vi "H5Fget_name.vi"(6 "error in (no error)":errorcluster, 9 "HDF5 Attr Ref":T1) -> (0 "error out":errorcluster, 2 "Name":string, 3 "HDF5 Attr Ref out":T1)   [LabVIEW 2017]
doc: "Retrieves name of file to which object belongs."
uses:
  <vilib>/UPVI/lvhdf5/library.llb/HDF5 Ref.ctl
  <vilib>/UPVI/lvhdf5/hdf5.dll
panel:
  # "LVHDF5 Toolkit\nCopyright (c) 2005-2013 by Jason D. Sommerville\nCopyright (c) 2014 by UPVI, LLC.\n\nThis use and distribution of this file is governed by the terms found in \nLICENSE.txt distributed with this toolkit and installed at\n <user.lib>\\_lvhdf5\\LICENSE.txt"
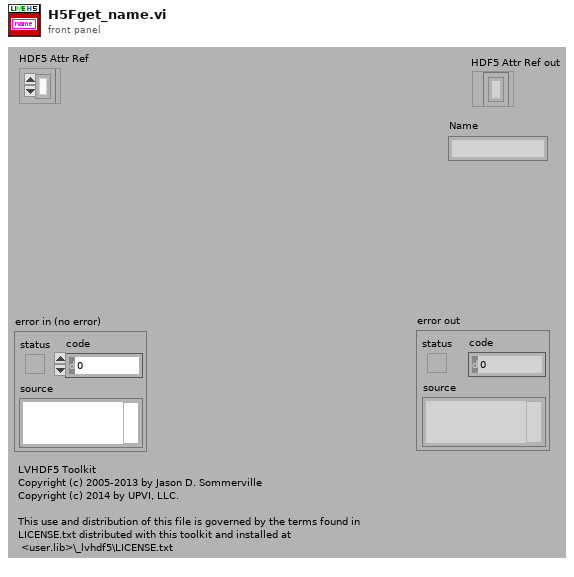
[diagram p1: front panel]
types:
  T1 = typedef "HDF5 Ref.ctl" = refnum<k1>
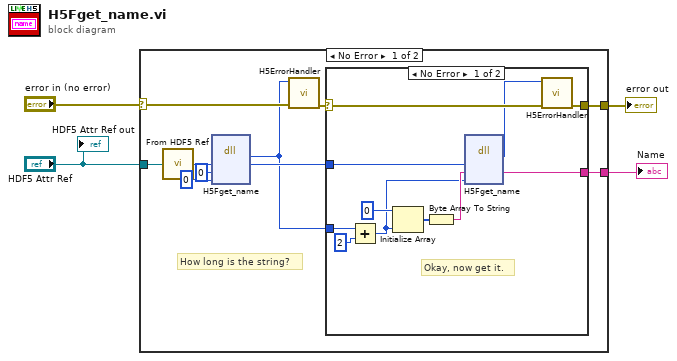
[diagram p0: block diagram]
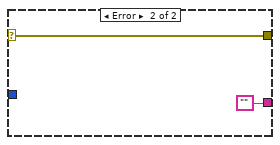
[diagram p2: hidden frame]
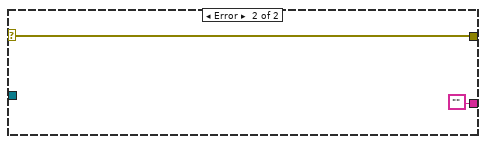
[diagram p3: hidden frame]
diagram:
  n1 = case shown="No Error" "error in (no error)" {
    selector: "error in (no error)" -> [w12 w29]
    tunnel: [w8 w29] -> w2
    tunnel: "HDF5 Attr Ref" -> [w14 _]
    tunnel: [w9 ""] -> w1
    frame No Error {
      # "How long is the string?"
      n2 = call <vilib>:"From HDF5 Ref.vi"("HDF5 Ref"=w14) -> ("I32"=w13:i32)
      n3 = dll-call lib="C:/Program Files/National Instruments/LabVIEW 2017/vi.lib/UPVI/lvhdf5/hdf5.dll" fn="H5Fget_name"("obj_id"=w13, "name"=0, "size"=u32 0) -> ("return type"=w7:u64, "obj_id"=w10:i32)  [unwired: 5 in, 2 out]
      n4 = call <vilib>:"H5ErrorHandler.vi"("error in (no error)"=w12, "herr_t"=w7) -> ("error out"=w11:errorcluster)  [unwired: 3 in, 4 out]
      n5 = case shown="No Error" w11 {
        selector: w11 -> [w23 w26]
        tunnel: w7 -> [w21 _]
        tunnel: w10 -> [w17 _]
        tunnel: [w22 w26] -> w8
        tunnel: [w15 ""] -> w9
        frame No Error {
          # "Okay, now get it."
          n6 = Add(x=w21, y=2) -> (x+y=w16:u64)
          n7 = Initialize Array(u8 0, w16) -> (w24:u8[])
          n8 = Byte Array To String(unsigned byte array=w24) -> (string=w18:string)
          n9 = dll-call lib="C:/Program Files/National Instruments/LabVIEW 2017/vi.lib/UPVI/lvhdf5/hdf5.dll" fn="H5Fget_name"("obj_id"=w17, "name"=w18, "size"=w16) -> ("return type"=w19:i64, "name"=w15:string)  [unwired: 5 in, 2 out]
          n10 = call <vilib>:"H5ErrorHandler.vi"("error in (no error)"=w23, "herr_t"=w19) -> ("error out"=w22:errorcluster)  [unwired: 3 in, 4 out]
        }
        frame Error {
        }
      }
    }
    frame Error {
    }
  }
  "error out" <- w2
  "Name" <- w1
  "HDF5 Attr Ref out" <- "HDF5 Attr Ref"
